vi "Better Steer Angle.vi"(0 "Current Angle":dbl(knob)=41.7137932364482 scale=0.0..360.0, 2 "Set Point":dbl(knob)=41.7137932364482 scale=0.0..360.0) -> (3 "Better Angle":dbl(knob)=41.7137932364482 scale=0.0..360.0, 4 "Degres To Travel":dbl, 5 "Encoder Count to Move":dbl, 6 "Flip motors?":bool)   [LabVIEW 2018]
uses:
  <vilib>/Analysis/coordinate.llb/Angle Units.ctl
  <vilib>/Analysis/coordinate.llb/Angle Range (Degree).ctl
  <vilib>/Analysis/coordinate.llb/Wrap Angle (scalar).vi
  <vilib>/Analysis/NI_AAL_Angle.lvlib
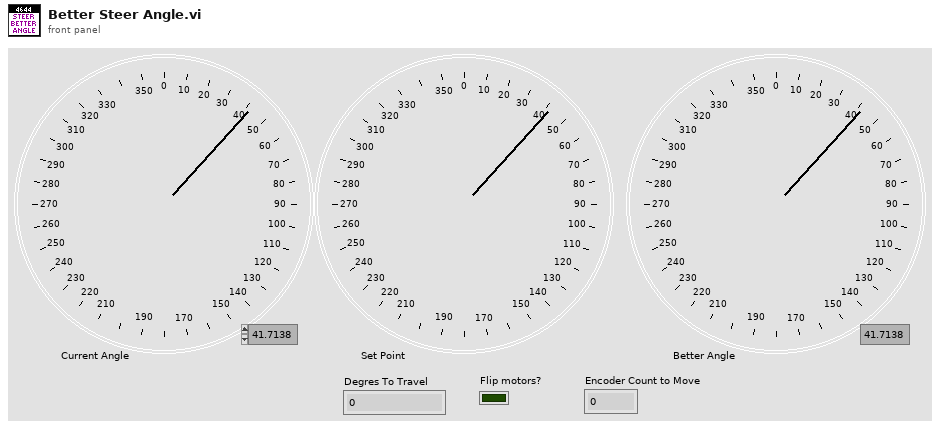
[diagram p1: front panel]
types:
  T1 = typedef "NI_AAL_Angle.lvlib/Angle Range (Degree).ctl" = u16
  T2 = typedef "NI_AAL_Angle.lvlib/Angle Units.ctl" = i32
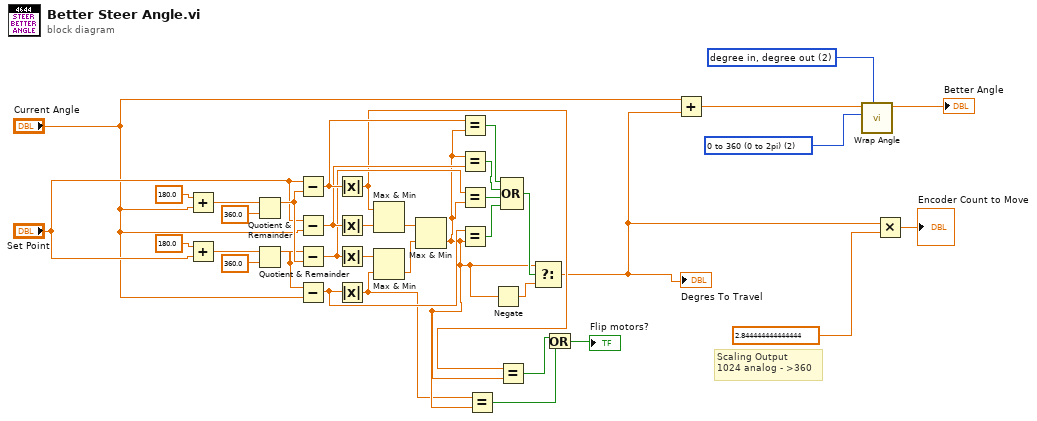
[diagram p0: block diagram]
diagram:
  w4 = T1 2 items=["none", "-180 to 180 (-pi to pi)", "0 to 360 (0 to 2pi)"] ("angle range")
  w5 = T2 2 items=["radian in, radian out", "radian in, degree out", "degree in, degree out", "degree in, radian out"] ("angle units")
  # "Scaling Output\n1024 analog - >360"
  n1 = Add(x=180.0, y="Current Angle") -> (x+y=w32:dbl)
  n2 = Add(x=180.0, y="Set Point") -> (x+y=w35:dbl)
  n3 = Quotient & Remainder(x=w32, y=360.0) -> (x-y*floor(x/y)=w31:dbl)  [unwired: 1 out]
  n4 = Quotient & Remainder(x=w35, y=360.0) -> (x-y*floor(x/y)=w25:dbl)  [unwired: 1 out]
  n5 = Subtract(x="Set Point", y=w31) -> (x-y=w20:dbl)
  n6 = Subtract(x="Set Point", y="Current Angle") -> (x-y=w19:dbl)
  n7 = Subtract(x=w25, y=w31) -> (x-y=w18:dbl)
  n8 = Subtract(x=w25, y="Current Angle") -> (x-y=w17:dbl)
  n9 = Absolute Value(x=w20) -> (abs(x)=w13:dbl)
  n10 = Absolute Value(x=w19) -> (abs(x)=w12:dbl)
  n11 = Absolute Value(x=w18) -> (abs(x)=w11:dbl)
  n12 = Absolute Value(x=w17) -> (abs(x)=w10:dbl)
  n13 = Max & Min(x=w13, y=w12) -> (min(x,y)=w29:dbl)  [unwired: 1 out]
  n14 = Max & Min(x=w11, y=w10) -> (min(x,y)=w30:dbl)  [unwired: 1 out]
  n15 = Max & Min(x=w29, y=w30) -> (min(x,y)=w16:dbl)  [unwired: 1 out]
  n16 = Equal?(x=w20, y=w16) -> (x = y?=w21:bool)
  n17 = Equal?(x=w16, y=w19) -> (x = y?=w26:bool)
  n18 = Equal?(x=w18, y=w16) -> (x = y?=w24:bool)
  n19 = Equal?(x=w17, y=w16) -> (x = y?=w22:bool)
  n20 = Equal?(x=w10, y=w16) -> (x = y?=w14:bool)
  n21 = Negate(x=w16) -> (-x=w27:dbl)
  n22 = Equal?(x=w13, y=w16) -> (x = y?=w15:bool)
  n23 = Compound Arithmetic op=OR(w21, w26, w24, w22) -> (w28:bool)
  n24 = Select(t=w16, s=w28, f=w27) -> (s? t:f=w2:dbl)
  "Degres To Travel" <- w2
  n25 = Or(x=w15, y=w14) -> (x .or. y?=→"Flip motors?":bool)
  n26 = Add(x="Current Angle", y=w2) -> (x+y=w8:dbl)
  n27 = call-poly <vilib>:"Wrap Angle.vi"("angle units"=w5, "angle range"=w4, "angle in"=w8) -> ("angle out"=→"Better Angle":dbl)  [unwired: 7 in, 1 out]
  n28 = Multiply(x=w2, y=2.844444444444444) -> (x*y=→"Encoder Count to Move":dbl)
